vi "Local Variables.vi"() -> ()   [LabVIEW 2012]
panel:
  in  "Stop Button":bool
  out "Chart 2":dbl(graph)
  out "Chart 1":dbl(graph)
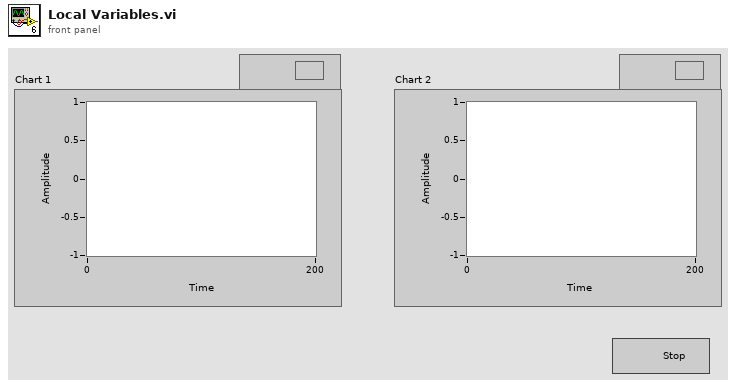
[diagram p1: front panel]
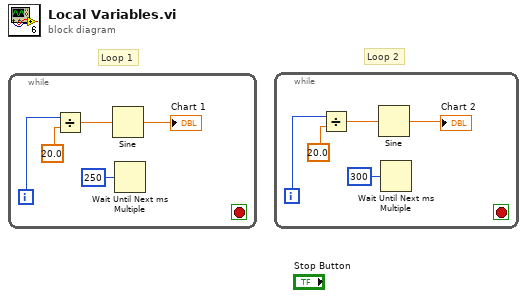
[diagram p0: block diagram]
diagram:
  # "Loop 1"
  # "Loop 2"
  n1 = while "Loop 1" {
    i -> [w5]
    stop <- _ stop-if-true
    n2 = Divide(x=w5, y=20.0) -> (x/y=w3:dbl)
    n3 = Sine(x=w3) -> (sin(x)=→"Chart 1":dbl)
    n4 = Wait Until Next ms Multiple(millisecond multiple=u32 250) -> ()  [unwired: 1 out]
  }
  n5 = while "Loop 2" {
    i -> [w10]
    stop <- _ stop-if-true
    n6 = Divide(x=w10, y=20.0) -> (x/y=w8:dbl)
    n7 = Sine(x=w8) -> (sin(x)=→"Chart 2":dbl)
    n8 = Wait Until Next ms Multiple(millisecond multiple=u32 300) -> ()  [unwired: 1 out]
  }
